vi "Approach Parametric Position.vi"(6 "Robot\nDimensions":cluster{}, 7 "Points":dbl[][](array[numeric]), 8 "Initial Forearm\nAngle":dbl format="%#_13g", 9 "Initial Backarm\nAngle":dbl format="%#_13g", 10 "Initial Parametric\nValue":dbl format="%#_13g", 11 "New Parametric\nValue":dbl) -> (0 "Next Forearm\nAngle":dbl, 1 "Next Backarm\nAngle":dbl, 3 "Next Parametric\nValue":dbl)   [LabVIEW 2017]
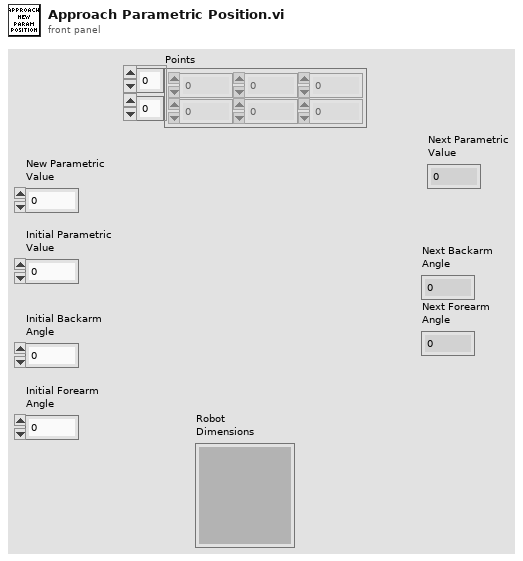
[diagram p1: front panel]
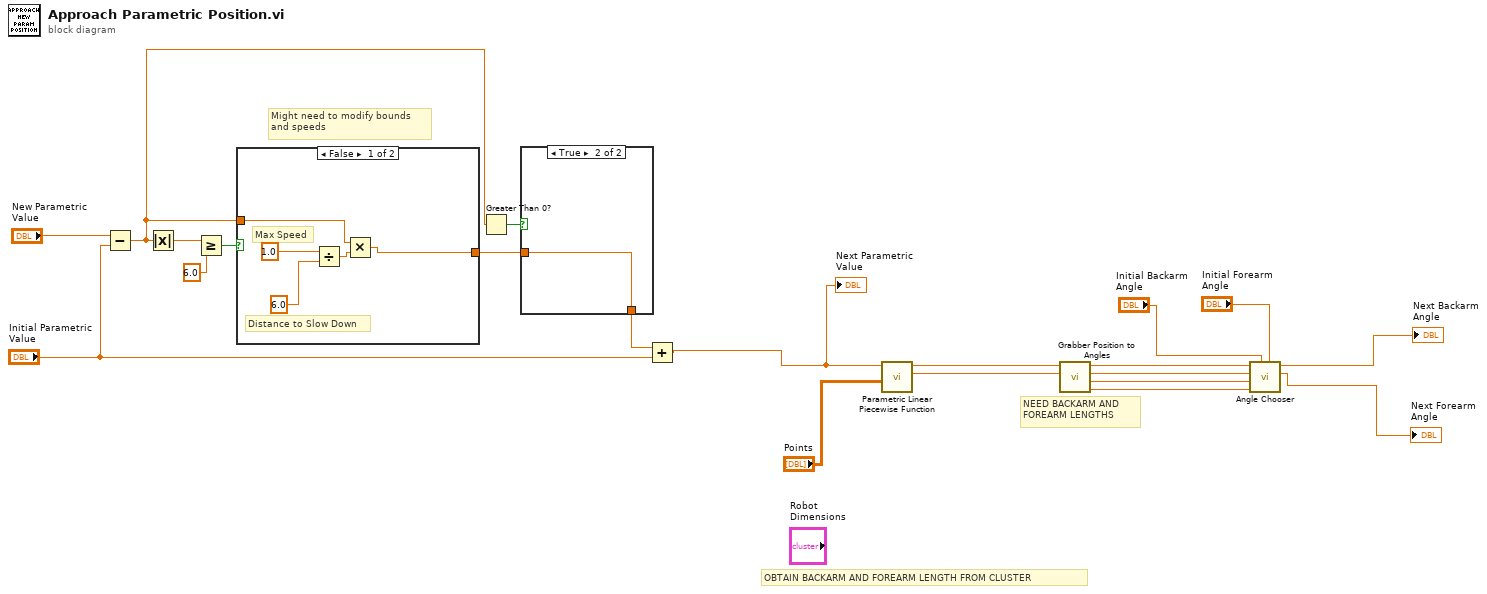
[diagram p0: block diagram]
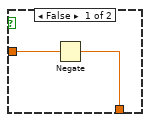
[diagram p2: hidden frame]
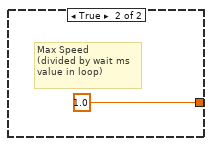
[diagram p3: hidden frame]
diagram:
  # "NEED BACKARM AND\nFOREARM LENGTHS"
  # "OBTAIN BACKARM AND FOREARM LENGTH FROM CLUSTER"
  # "Might need to modify bounds\nand speeds"
  n1 = Subtract(x="New Parametric\nValue", y="Initial Parametric\nValue") -> (x-y=w2:dbl)
  n2 = Absolute Value(x=w2) -> (abs(x)=w1:dbl)
  n3 = Greater Or Equal?(x=w1, y=6.0) -> (x >= y?=w7:bool)
  n4 = case shown="False" w7 {
    tunnel: [w26 1.0] -> w4
    tunnel: w2 -> [w25 _]
    frame False {
      # "Distance to Slow Down"
      # "Max Speed"
      n5 = Divide(x=1.0, y=6.0) -> (x/y=w24:dbl)
      n6 = Multiply(x=w25, y=w24) -> (x*y=w26:dbl)
    }
    frame True {
      # "Max Speed\n(divided by wait ms\nvalue in loop)"
    }
  }
  n7 = Greater Than 0?(x=w2) -> (x > 0?=w5:bool)
  n8 = case shown="True" w5 {
    tunnel: w4 -> [w29 w30]
    tunnel: [w28 w30] -> w3
    frame False {
      n9 = Negate(x=w29) -> (-x=w28:dbl)
    }
    frame True {
    }
  }
  n10 = Add(x=w3, y="Initial Parametric\nValue") -> (x+y=w10:dbl)
  "Next Parametric\nValue" <- w10
  n11 = call "Parametric Linear Piecewise Function.vi"("Points"="Points", "Parametric\nValue"=w10) -> ("Y Position"=w14:dbl, "X Position"=w15:dbl)  [unwired: 8 in]
  n12 = call "Grabber Position to Angles.vi"("Y Initial"=w14, "X Initial"=w15) -> ("Forearm Angle\nDegrees 2"=w18:dbl, "Backarm Angle\nDegrees 2"=w19:dbl, "Forearm Angle\nDegrees 1"=w20:dbl, "Backarm Angle\nDegrees 1"=w21:dbl)  [unwired: 6 in]
  n13 = call "Angle Chooser.vi"("Forearm Angle Initial"="Initial Forearm\nAngle", "Backarm Angle Initial"="Initial Backarm\nAngle", "Forearm Angle 2"=w18, "Backarm Angle 2"=w19, "Forearm Angle 1"=w20, "Backarm Angle 1"=w21) -> ("final Forearm Angle"=→"Next Forearm\nAngle":dbl, "final Backarm Angle"=→"Next Backarm\nAngle":dbl)  [unwired: 4 in]
